vi "Run Framework.vi"(5 "components directory":path, 7 "framework options":T18={"FIFO Options"={"Infinite Timeouts"=FALSE}, "Thread Options"={"Show FP On Call"=TRUE, "Close FP After Call"=TRUE, "Allow Debugging"=TRUE}, "Plugin Options"={"Default Components"=TRUE}, "Performance Options"={"Measure Period"=TRUE, "Measure Rx/Tx Duration"=TRUE}, "Data Server Options"={"Enable Data Server"=FALSE, "Period"=50}} {"Data Server Options"."Period" format="%d ms"}, 8 "error in (no error)":errorcluster, 9 "thread settings":cluster{"Processor":i32, "Priority":i32}={"Processor"=-2, "Priority"=100}, 10 "framework configuration":T2, 11 "user interface pointers (null)":T1) -> (0 "error out":errorcluster)   [LabVIEW 2020]
uses:
  Includes/DSF Core.lvlibp/Classes/Framework/Framework Options.ctl
  Includes/DSF Core.lvlibp/Typedefs/DSF FIFO Options.ctl
  Includes/DSF Core.lvlibp/Classes/Thread/Thread Options.ctl
  Includes/DSF Core.lvlibp/Typedefs/DSF Plugin Options.ctl
  Includes/DSF Core.lvlibp/Typedefs/DSF Performance Options.ctl
  Includes/DSF Core.lvlibp/Classes/Framework/Data Server Options.ctl
  Includes/DSF Core.lvlibp/Typedefs/DSF Engine Framework Configuration.ctl
  Includes/DSF Core.lvlibp/Typedefs/DSF Engine Plugin Configuration.ctl
  Includes/DSF Core.lvlibp/Typedefs/Core Plugin Configuration.ctl
  Includes/DSF Core.lvlibp/Typedefs/DSF Timing Info.ctl
  Includes/DSF Core.lvlibp/Typedefs/DSF Settings Info.ctl
  Includes/DSF Core.lvlibp/Typedefs/DSF Engine Plugin Thread Configuration.ctl
  Includes/DSF Core.lvlibp/Typedefs/Core Thread Configuration.ctl
  Includes/DSF Core.lvlibp/Typedefs/DSF Engine Transfer Group Configuration.ctl
  Includes/DSF Core.lvlibp/Typedefs/Core Group Configuration.ctl
  Includes/DSF Core.lvlibp/Typedefs/DSF Direction.ctl
  Includes/DSF Core.lvlibp/Typedefs/DSF Timeout Behavior.ctl
  Includes/DSF Core.lvlibp/Typedefs/DSF Engine Transfer Configuration.ctl
  Includes/DSF Core.lvlibp/Typedefs/Core Transfer Configuration.ctl
  Includes/DSF Core.lvlibp/Typedefs/DSF Engine Channel Configuration.ctl
  Includes/DSF Core.lvlibp/Typedefs/Core Channel Configuration.ctl
  Includes/DSF Core.lvlibp/Typedefs/DSF Data Type.ctl
  SubVIs/UI Pointers.ctl
  <vilib>/NI/Memory Manager/Classes/Pointer/Pointer.lvclass
  <vilib>/NI/Memory Manager/Classes/Pointer/Pointer.lvclass/Pointer.ctl
  <vilib>/Platform/TimedLoop/XDataNode/timing_clust.ctl
  <vilib>/Platform/TimedLoop/XDataNode/nitl_modes.ctl
  <vilib>/Platform/TimedLoop/XDataNode/wakeup.ctl
  <vilib>/NI/Memory Manager/Classes/Pointer/Write U32.vi
  <vilib>/NI/Memory Manager/Classes/Pointer/Read U32.vi
  <vilib>/NI/Memory Manager/Classes/Pointer/Read I32.vi
  <vilib>/NI/Memory Manager/Classes/Pointer/Read Bool.vi
  <vilib>/NI/Memory Manager/Classes/Pointer/Write Bool.vi
  <vilib>/NI/Memory Manager/Classes/Pointer/Write I32.vi
  <vilib>/NI/Memory Manager/Classes/Pointer/Set Address.vi
  <vilib>/NI/Memory Manager/Classes/Pointer/Set Size.vi
  <vilib>/NI/Memory Manager/Classes/Pointer/Set Internal.vi
  <vilib>/NI/Memory Manager/Classes/Pointer/Check Null Pointer.vi
  <vilib>/NI/Memory Manager/Classes/Pointer/Clear (No Check).vi
  <vilib>/NI/Memory Manager/Classes/Pointer/Check Length.vi
  <vilib>/NI/Memory Manager/Classes/Pointer/Write (No Check).vi
  <vilib>/NI/Memory Manager/Classes/Pointer/Write (No Check) U32.vi
  <vilib>/NI/Memory Manager/Classes/Pointer/Check Move.vi
  <vilib>/NI/Memory Manager/Classes/Pointer/Read (No Check).vi
  <vilib>/NI/Memory Manager/Classes/Pointer/Read (No Check) U32.vi
  <vilib>/NI/Memory Manager/Classes/Pointer/Read (No Check) I32.vi
  <vilib>/NI/Memory Manager/Classes/Pointer/Read (No Check) Bool.vi
  <vilib>/NI/Memory Manager/Classes/Pointer/Write (No Check) Bool.vi
  <vilib>/NI/Memory Manager/Classes/Pointer/Write (No Check) I32.vi
  <vilib>/NI/Memory Manager/Classes/Pointer/Get Internal.vi
  <vilib>/NI/Memory Manager/Classes/Pointer/Errors.vi
  <vilib>/NI/Memory Manager/Classes/Pointer/Zone.vi
  <vilib>/NI/Memory Manager/Classes/Pointer/Null Pointer.vi
  <vilib>/NI/Memory Manager/Classes/Pointer/Check Bounds (Pointer).vi
  <vilib>/NI/Memory Manager/Classes/Pointer/Check Count.vi
  <vilib>/NI/Memory Manager/Classes/Pointer/Check Bounds (Power of 2).vi
  <vilib>/NI/Memory Manager/Classes/Pointer/Create Error.vi
  <vilib>/NI/Memory Manager/Classes/Pointer/Out of Bounds.vi
  <vilib>/NI/Memory Manager/Classes/Pointer/Check Bounds.vi
  <vilib>/NI/Memory Manager/VIs/New Error Cluster.vi
  <vilib>/NI/Memory Manager/VIs/New Error Cluster (512B).vi
  <vilib>/NI/Memory Manager/VIs/Set Error Status.vi
  <vilib>/NI/Memory Manager/VIs/Set Error Code.vi
  <vilib>/NI/Memory Manager/VIs/Set Error Source.vi
  <vilib>/NI/Memory Manager/Constants/Constants.vi
  <vilib>/NI/Memory Manager/Constants/Library Name.vi
  <vilib>/NI/Memory Manager/Classes/Pointer/Pointer Error Info.vi
  <vilib>/NI/Memory Manager/VIs/Write String to Source.vi
  <vilib>/NI/Memory Manager/Constants/Pointer Class Name.vi
  <vilib>/NI/Memory Manager/Classes/Pointer/Write Pointer Size to Error.vi
  <vilib>/NI/Memory Manager/VIs/Write Numeric to Source.vi
  <vilib>/NI/Memory Manager/VIs/Write Numeric Scalar to Source (Base10 U64).vi
  <vilib>/NI/Memory Manager/Classes/Pointer/Check Bounds (Buffer).vi
  <vilib>/NI/Memory Manager/Classes/Pointer/Buffer Underflow.vi
  Includes/DSF Core.lvlibp/Classes/Framework/Framework.lvclass
  <vilib>/platform/TimedLoop/XDataNode/XDataNode.xnode
  <vilib>/Platform/TimedLoop/XDataNode/XDNodeRunTimeDep.lvlib
  Includes/DSF Core.lvlibp/Classes/Configuration/Core/Framework/Framework Configuration.lvclass
  Includes/DSF Core.lvlibp
  Includes/DSF Core.lvlibp/Classes/Thread/Thread.lvclass
  Includes/DSF Core.lvlibp/Classes/Configuration/Core/Plugin/Plugin Configuration.lvclass
  Includes/DSF Core.lvlibp/Classes/Configuration/Core/Thread/Thread Configuration.lvclass
  Includes/DSF Core.lvlibp/Classes/Configuration/Core/Group/Group Configuration.lvclass
  Includes/DSF Core.lvlibp/Classes/Configuration/Core/Transfer/Transfer Configuration.lvclass
  Includes/DSF Core.lvlibp/Classes/Configuration/Core/Channel/Channel Configuration.lvclass
panel:
  out "actual frequency":u32 format="%.0pHz"
  in  "target frequency":u32=100 format="%.0pHz"
  out "iteration":i32
  in  "stop":bool
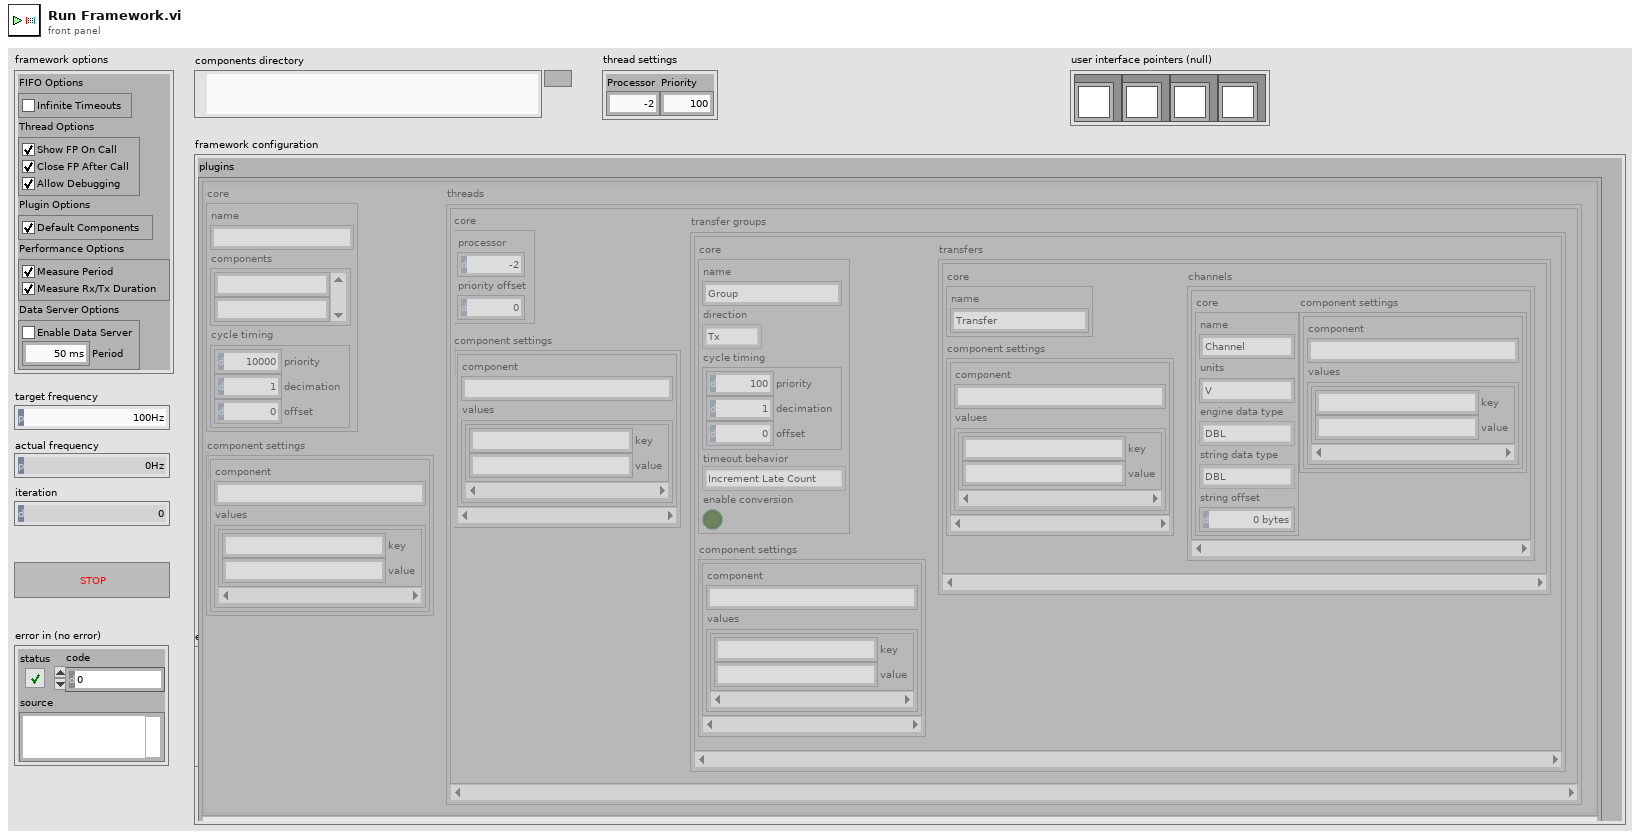
[diagram p1: front panel]
types:
  T1 = typedef "UI Pointers.ctl" = cluster{"Stop":refnum<class "Pointer.lvclass">, "Target Period":refnum<class "Pointer.lvclass">, "Actual Period":refnum<class "Pointer.lvclass">, "Iteration":refnum<class "Pointer.lvclass">}
  T2 = typedef "DSF Core.lvlibp/DSF Engine Framework Configuration.ctl" = cluster{"plugins":T3[]}
  T3 = typedef "DSF Core.lvlibp/DSF Engine Plugin Configuration.ctl" = cluster{"core":T4, "component settings":T6[], "threads":T7[]}
  T4 = typedef "DSF Core.lvlibp/Plugin Configuration.lvclass/Core Plugin Configuration.ctl" = cluster{"name":string, "components":string[], "cycle timing":T5}
  T5 = typedef "DSF Core.lvlibp/DSF Timing Info.ctl" = cluster{"priority":u64, "decimation":u64, "offset":u64}
  T6 = typedef "DSF Core.lvlibp/DSF Settings Info.ctl" = cluster{"component":string, "values":cluster{"key":string, "value":string}[]}
  T7 = typedef "DSF Core.lvlibp/DSF Engine Plugin Thread Configuration.ctl" = cluster{"core":T8, "component settings":T6[], "transfer groups":T9[]}
  T8 = typedef "DSF Core.lvlibp/Thread Configuration.lvclass/Core Thread Configuration.ctl" = cluster{"processor":i32, "priority offset":i16}
  T9 = typedef "DSF Core.lvlibp/DSF Engine Transfer Group Configuration.ctl" = cluster{"core":T10, "component settings":T6[], "transfers":T13[]}
  T10 = typedef "DSF Core.lvlibp/Group Configuration.lvclass/Core Group Configuration.ctl" = cluster{"name":string, "direction":T11, "cycle timing":T5, "timeout behavior":T12, "enable conversion":bool}
  T11 = typedef "DSF Core.lvlibp/DSF Direction.ctl" = enum8{"Tx", "Rx"}
  T12 = typedef "DSF Core.lvlibp/DSF Timeout Behavior.ctl" = enum8{"Increment Late Count", "Throw Error"}
  T13 = typedef "DSF Core.lvlibp/DSF Engine Transfer Configuration.ctl" = cluster{"core":T14, "component settings":T6[], "channels":T15[]}
  T14 = typedef "DSF Core.lvlibp/Transfer Configuration.lvclass/Core Transfer Configuration.ctl" = cluster{"name":string}
  T15 = typedef "DSF Core.lvlibp/DSF Engine Channel Configuration.ctl" = cluster{"core":T16, "component settings":T6[]}
  T16 = typedef "DSF Core.lvlibp/Channel Configuration.lvclass/Core Channel Configuration.ctl" = cluster{"name":string, "units":string, "engine data type":T17, "string data type":T17, "string offset":u64}
  T17 = typedef "DSF Core.lvlibp/DSF Data Type.ctl" = enum8{"Bool", "SGL", "DBL", "I8", "I16", "I32", "I64", "U8", "U16", "U32", "U64"}
  T18 = typedef "DSF Core.lvlibp/Framework.lvclass/Framework Options.ctl" = cluster{"FIFO Options":T19, "Thread Options":T20, "Plugin Options":T21, "Performance Options":T22, "Data Server Options":T23}
  T19 = typedef "DSF Core.lvlibp/Framework.lvclass/DSF FIFO Options.ctl" = cluster{"Infinite Timeouts":bool}
  T20 = typedef "DSF Core.lvlibp/Thread.lvclass/Thread Options.ctl" = cluster{"Show FP On Call":bool, "Close FP After Call":bool, "Allow Debugging":bool}
  T21 = typedef "DSF Core.lvlibp/Framework.lvclass/DSF Plugin Options.ctl" = cluster{"Default Components":bool}
  T22 = typedef "DSF Core.lvlibp/DSF Performance Options.ctl" = cluster{"Measure Period":bool, "Measure Rx/Tx Duration":bool}
  T23 = typedef "DSF Core.lvlibp/Framework.lvclass/Data Server Options.ctl" = cluster{"Enable Data Server":bool, "Period":u32}
  T24 = typedef "XDNodeRunTimeDep.lvlib/timing_clust.ctl" = cluster{"Expected End [f-1]":u64, "Actual End [f-1]":u64, "Finished Late? [f-1]":bool, "Expected End [i-1]":u64, "Actual End [i-1]":u64, "Finished Late? [i-1]":bool, "Expected Start [i]":u64, "Actual Start [i]":u64, "Expected Start [f]":u64, "Actual Start [f]":u64, "Source Name":string, "Structure Name":string, "Period":i64, "Deadline":i64, "Offset":i64, "Start":i64, "Priority":i32, "Timeout":i32, "Mode":T25, "Wakeup Reason":T26, "Error":errorcluster, "Source Type":string, "Secondary Source Type":string, "Global End Time":u64, "Global Start Time":u64, "Frame Duration":u64, "Iteration Duration":u64, "Assigned CPU":i32, "I/O Scan Engine Mode":u32}
  T25 = typedef "XDNodeRunTimeDep.lvlib/nitl_modes.ctl" = enum32{"No Change", "Process missed periods, maintain original phase", "Discard missed periods, maintain original phase", "Process missed periods, ignore original phase", "Discard missed periods, ignore original phase"}
  T26 = typedef "XDNodeRunTimeDep.lvlib/wakeup.ctl" = enum32{"Normal", "Aborted", "Asynchronous wakeup", "Timing source error", "Timed loop error", "Timeout"}
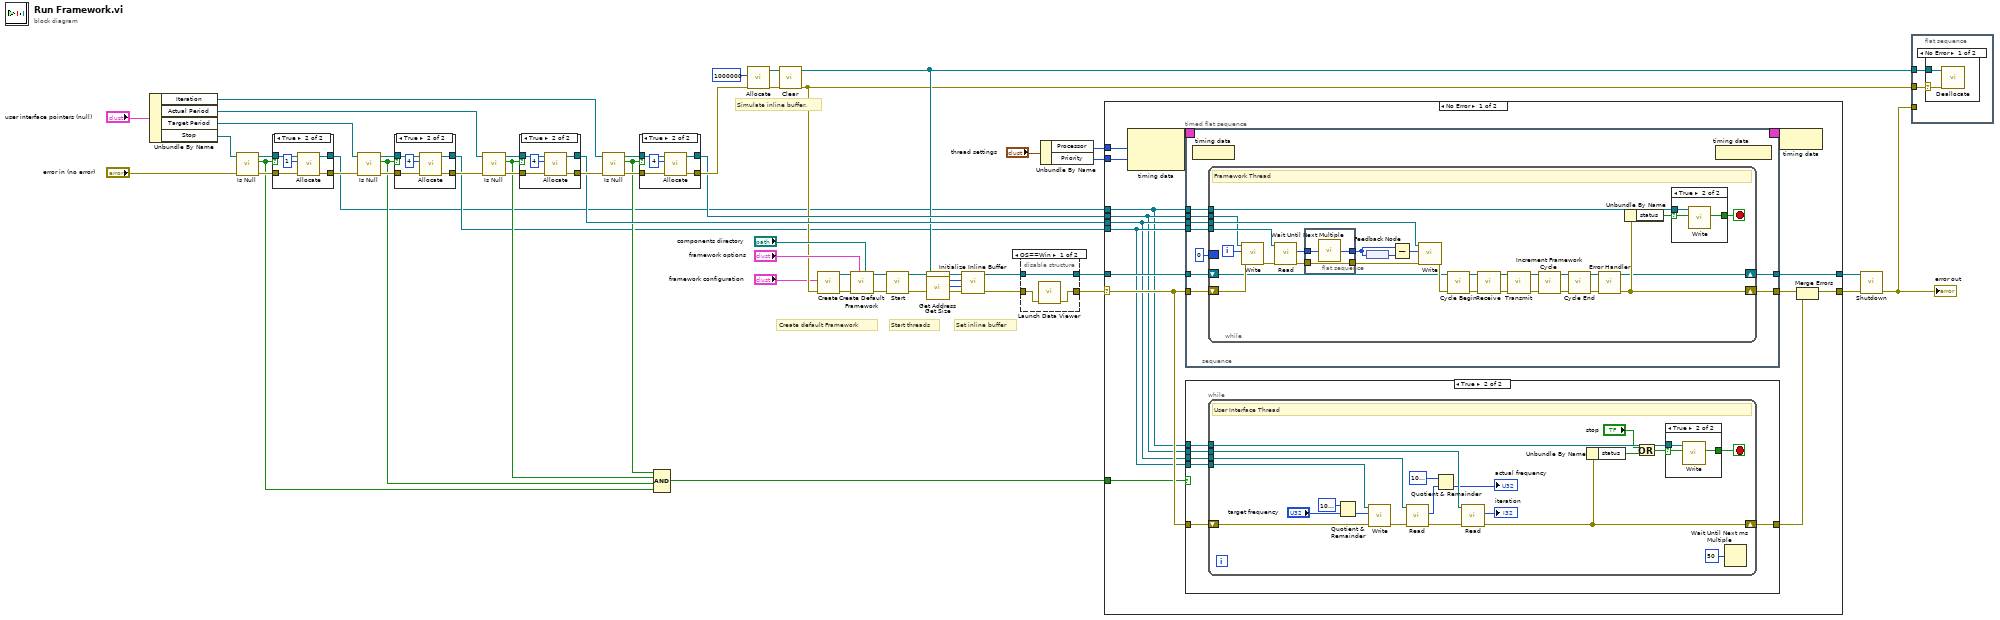
[diagram p0: block diagram]
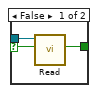
[diagram p5: hidden frame]
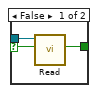
[diagram p6: hidden frame]
diagram:
  # "Set inline buffer"
  # "Start threads"
  # "Create default Framework"
  # "Simulate inline buffer."
  n1 = Unbundle By Name("user interface pointers (null)") -> ("Iteration"=w21:refnum<class "Pointer.lvclass">, "Actual Period"=w25:refnum<class "Pointer.lvclass">, "Target Period"=w29:refnum<class "Pointer.lvclass">, "Stop"=w35:refnum<class "Pointer.lvclass">)
  n2 = call <vilib>:"Is Null.vi"("error in (no error)"="error in (no error)", "Pointer in"=w35) -> ("error out"=w33:errorcluster, "null?"=w11:bool, "Pointer out"=w34:refnum<class "Pointer.lvclass">)  [unwired: 7 in]
  n3 = case shown="True" w11 {
    tunnel: w34 -> [w55 w59]
    tunnel: w33 -> [w54 w58]
    tunnel: [w55 w57] -> w1
    tunnel: [w54 w56] -> w30
    frame False {
    }
    frame True {
      n4 = call <vilib>:"Allocate.vi"("error in (no error)"=w58, "size"=u64 1, "Pointer type"=w59) -> ("error out"=w56:errorcluster, "Pointer out"=w57:refnum<class "Pointer.lvclass">)  [unwired: 7 in]
    }
  }
  n5 = call <vilib>:"Is Null.vi"("error in (no error)"=w30, "Pointer in"=w29) -> ("error out"=w31:errorcluster, "null?"=w10:bool, "Pointer out"=w32:refnum<class "Pointer.lvclass">)  [unwired: 7 in]
  n6 = case shown="True" w10 {
    tunnel: w32 -> [w62 w66]
    tunnel: w31 -> [w61 w65]
    tunnel: [w62 w64] -> w2
    tunnel: [w61 w63] -> w26
    frame False {
    }
    frame True {
      n7 = call <vilib>:"Allocate.vi"("error in (no error)"=w65, "size"=u64 4, "Pointer type"=w66) -> ("error out"=w63:errorcluster, "Pointer out"=w64:refnum<class "Pointer.lvclass">)  [unwired: 7 in]
    }
  }
  n8 = call <vilib>:"Is Null.vi"("error in (no error)"=w26, "Pointer in"=w25) -> ("error out"=w27:errorcluster, "null?"=w9:bool, "Pointer out"=w28:refnum<class "Pointer.lvclass">)  [unwired: 7 in]
  n9 = case shown="True" w9 {
    tunnel: w28 -> [w69 w73]
    tunnel: w27 -> [w68 w72]
    tunnel: [w69 w71] -> w17
    tunnel: [w68 w70] -> w22
    frame False {
    }
    frame True {
      n10 = call <vilib>:"Allocate.vi"("error in (no error)"=w72, "size"=u64 4, "Pointer type"=w73) -> ("error out"=w70:errorcluster, "Pointer out"=w71:refnum<class "Pointer.lvclass">)  [unwired: 7 in]
    }
  }
  n11 = call <vilib>:"Is Null.vi"("error in (no error)"=w22, "Pointer in"=w21) -> ("error out"=w23:errorcluster, "null?"=w8:bool, "Pointer out"=w24:refnum<class "Pointer.lvclass">)  [unwired: 7 in]
  n12 = case shown="True" w8 {
    tunnel: w24 -> [w76 w80]
    tunnel: w23 -> [w75 w79]
    tunnel: [w76 w78] -> w18
    tunnel: [w75 w77] -> w20
    frame False {
    }
    frame True {
      n13 = call <vilib>:"Allocate.vi"("error in (no error)"=w79, "size"=u64 4, "Pointer type"=w80) -> ("error out"=w77:errorcluster, "Pointer out"=w78:refnum<class "Pointer.lvclass">)  [unwired: 7 in]
    }
  }
  n14 = Compound Arithmetic op=AND(w8, w9, w10, w11) -> (w7:bool)
  n15 = call <vilib>:"Allocate.vi"("error in (no error)"=w20, "size"=u64 1000000) -> ("error out"=w49:errorcluster, "Pointer out"=w46:refnum<class "Pointer.lvclass">)  [unwired: 8 in]
  n16 = call <vilib>:"Clear.vi"("error in (no error)"=w49, "Pointer in"=w46) -> ("error out"=w6:errorcluster, "Pointer out"=w16:refnum<class "Pointer.lvclass">)  [unwired: 8 in]
  n17 = call "Create.vi"("error in (no error)"=w6, "framework configuration"="framework configuration") -> ("error out"=w5:errorcluster, "Framework Configuration out"=w4:refnum<class "Framework Configuration.lvclass">)  [unwired: 8 in]
  n18 = call "Create Default Framework.vi"("components directory (default)"="components directory", "framework options"="framework options", "error in (no error)"=w5, "Framework Configuration"=w4) -> ("error out"=w41:errorcluster, "Framework"=w45:refnum<class "Framework.lvclass">)  [unwired: 6 in]
  n19 = call-dynamic "Start.vi"("error in (no error)"=w41, "Framework in"=w45) -> ("error out"=w44:errorcluster, "Framework out"=w53:refnum<class "Framework.lvclass">)  [unwired: 8 in]
  n20 = call <vilib>:"Get Address.vi"("Pointer in"=w16) -> ("address"=w47:u64)  [unwired: 9 in, 1 out]
  n21 = call <vilib>:"Get Size.vi"("Pointer in"=w16) -> ("size"=w48:u64)  [unwired: 9 in, 1 out]
  n22 = call "Initialize Inline Buffer.vi"("error in (no error)"=w44, "size"=w48, "address"=w47, "Framework in"=w53) -> ("error out"=w42:errorcluster, "Framework out"=w43:refnum<class "Framework.lvclass">)  [unwired: 6 in]
  n23 = disable-structure shown="OS==Win" {
    disable-tunnel: [w84 w86] -> w39
    disable-tunnel: [w82 w85] -> w19
    disable-tunnel: w43 -> [w84 w86]
    disable-tunnel: w42 -> [w83 w85]
    frame condition #0 (active) {
      n24 = call "Launch Data Viewer.vi"("error in (no error)"=w83) -> ("error out"=w82:errorcluster)  [unwired: 10 in]
    }
    frame condition #1 {
    }
  }
  n25 = Unbundle By Name("thread settings") -> ("Processor"=w13:i32, "Priority"=w14:i32)
  n26 = case shown="No Error" w19 {
    selector: w19 -> [w101 w197]
    tunnel: [w94 w197] -> w52
    tunnel: w39 -> [w100 w198]
    tunnel: [w98 w198] -> w51
    tunnel: w1 -> [w91 _]
    tunnel: w2 -> [w99 _]
    tunnel: w17 -> [w93 _]
    tunnel: w18 -> [w92 _]
    tunnel: w13 -> [w90 _]
    tunnel: w14 -> [w89 _]
    tunnel: w7 -> [w88 _]
    frame No Error {
      n27 = node-c288(w90, w89) -> (w97:T24)
      n28 = timed-sequence {
        timing: w97 -> [_]
        timing-out: [_] -> w96
        tunnel: w100 -> [w142]
        tunnel: w101 -> [w141]
        tunnel: [w140] -> w98
        tunnel: [w139] -> w95
        tunnel: w91 -> [w138]
        tunnel: w99 -> [w137]
        tunnel: w93 -> [w136]
        tunnel: w92 -> [w135]
        n29 = timed-flat-sequence {
          tunnel: w142 -> [w151]
          tunnel: w141 -> [w150]
          tunnel: [w149] -> w140
          tunnel: [w148] -> w139
          tunnel: w138 -> [w147]
          tunnel: w137 -> [w146]
          tunnel: w136 -> [w145]
          tunnel: w135 -> [w144]
          n30 = node-c288() -> ()  [unwired: 1 in]
          n31 = while {
            shift-right: [w170] -> w149
            shift-left: w151 -> [w155]
            tunnel: w147 -> [w178]
            shift-right: [w173] -> w148
            shift-left: w150 -> [w159]
            tunnel: w146 -> [w171]
            tunnel: w145 -> [w161]
            tunnel: w144 -> [w158]
            border: u32 0 ("Tick Count(uSec)") -> [_]
            i -> [w163]
            stop <- w177 stop-if-true
            # "Framework Thread"
            n32 = call-poly <vilib>:"Write.vi"("error in (no error)"=w159, "value"=w163, "Pointer in"=w158) -> ("error out"=w160:errorcluster)  [unwired: 5 in, 3 out]
            n33 = call-poly <vilib>:"Read.vi"("error in (no error)"=w160, "Pointer in"=w171) -> ("error out"=w157:errorcluster, "value out"=w172:u32)  [unwired: 6 in, 2 out]
            n34 = flat-sequence {
              tunnel: w172 -> [w183]
              tunnel: [w182] -> w154
              tunnel: w157 -> [w181]
              tunnel: [w181] -> w156
              frame #0 {
                n35 = call "Wait Until Next Multiple"("Count(uSec)"=w183) -> ("Tick Count(uSec)"=w182:u32)
              }
            }
            n36 = feedback-in #1(w154) -> ()
            n37 = feedback #1() -> (w152:u32)
            n38 = Subtract(x=w154, y=w152) -> (x-y=w153:u32)
            n39 = call-poly <vilib>:"Write.vi"("error in (no error)"=w156, "value"=w153, "Pointer in"=w161) -> ("error out"=w162:errorcluster)  [unwired: 5 in, 3 out]
            n40 = call "Cycle Begin.vi"("error in (no error)"=w162, "Framework in"=w155) -> ("error out"=w175:errorcluster, "Framework out"=w176:refnum<class "Framework.lvclass">)  [unwired: 8 in]
            n41 = call "Receive.vi"("error in"=w175, "framework in"=w176) -> ("error out"=w180:errorcluster, "framework out"=w179:refnum<class "Framework.lvclass">)  [unwired: 8 in]
            n42 = call "Transmit.vi"("error in"=w180, "framework in"=w179) -> ("error out"=w169:errorcluster, "framework out"=w168:refnum<class "Framework.lvclass">)  [unwired: 8 in]
            n43 = call "Increment Framework Cycle.vi"("error in (no error)"=w169, "Framework in"=w168) -> ("error out"=w166:errorcluster, "Framework out"=w167:refnum<class "Framework.lvclass">)  [unwired: 8 in]
            n44 = call "Cycle End.vi"("error in (no error)"=w166, "Framework in"=w167) -> ("error out"=w165:errorcluster, "Framework out"=w164:refnum<class "Framework.lvclass">)  [unwired: 8 in]
            n45 = call "Error Handler.vi"("error in (no error)"=w165, "Framework in"=w164) -> ("error out"=w173:errorcluster, "Framework out"=w170:refnum<class "Framework.lvclass">)  [unwired: 8 in]
            n46 = Unbundle By Name(w173) -> ("status"=w174:bool)
            n47 = case shown="True" w174 {
              selector: w174 -> [w185 w188]
              tunnel: w178 -> [w186 w189]
              tunnel: [w184 w187] -> w177
              frame False {
                n48 = call-poly <vilib>:"Read.vi"("value in"=w185, "Pointer in"=w186) -> ("value out"=w184:bool)  [unwired: 6 in, 3 out]
              }
              frame True {
                n49 = call-poly <vilib>:"Write.vi"("value"=w188, "Pointer in"=w189) -> ("value"=w187:bool)  [unwired: 6 in, 3 out]
              }
            }
          }
          n50 = node-c288() -> ()  [unwired: 1 out]
        }
      }
      n51 = case shown="True" w88 {
        tunnel: w101 -> [w102 w108]
        tunnel: w99 -> [_ w107]
        tunnel: [w102 w106] -> w87
        tunnel: w93 -> [_ w105]
        tunnel: w92 -> [_ w104]
        tunnel: w91 -> [_ w103]
        frame False {
        }
        frame True {
          n52 = while {
            tunnel: w103 -> [w128]
            shift-right: [w115] -> w106
            shift-left: w108 -> [w123]
            tunnel: w107 -> [w119]
            tunnel: w105 -> [w117]
            tunnel: w104 -> [w113]
            stop <- w127 stop-if-true
            # "User Interface Thread"
            n53 = Quotient & Remainder(x=u32 1000000 ("y"), y="target frequency") -> (floor(x/y)=w118:u32)  [unwired: 1 out]
            n54 = call-poly <vilib>:"Write.vi"("error in (no error)"=w123, "value"=w118, "Pointer in"=w119) -> ("error out"=w120:errorcluster)  [unwired: 5 in, 3 out]
            n55 = call-poly <vilib>:"Read.vi"("error in (no error)"=w120, "Pointer in"=w117) -> ("error out"=w116:errorcluster, "value out"=w109:u32)  [unwired: 6 in, 2 out]
            n56 = Quotient & Remainder(x=u32 1000000 ("y"), y=w109) -> (floor(x/y)=→"actual frequency":u32)  [unwired: 1 out]
            n57 = call-poly <vilib>:"Read.vi"("error in (no error)"=w116, "Pointer in"=w113) -> ("error out"=w115:errorcluster, "value out"=→"iteration":i32)  [unwired: 6 in, 2 out]
            n58 = Unbundle By Name(w115) -> ("status"=w125:bool)
            n59 = Or(x="stop", y=w125) -> (x .or. y?=w126:bool)
            n60 = case shown="True" w126 {
              selector: w126 -> [w130 w133]
              tunnel: w128 -> [w131 w134]
              tunnel: [w129 w132] -> w127
              frame False {
                n61 = call-poly <vilib>:"Read.vi"("value in"=w130, "Pointer in"=w131) -> ("value out"=w129:bool)  [unwired: 6 in, 3 out]
              }
              frame True {
                n62 = call-poly <vilib>:"Write.vi"("value"=w133, "Pointer in"=w134) -> ("value"=w132:bool)  [unwired: 6 in, 3 out]
              }
            }
            n63 = Wait Until Next ms Multiple(millisecond multiple=u32 50) -> ()  [unwired: 1 out]
          }
        }
      }
      n64 = node-c288(w96) -> ()
      n65 = Merge Errors(w95, w87) -> (w94:errorcluster)
    }
    frame Error {
    }
  }
  n66 = call-dynamic "Shutdown.vi"("error in (no error)"=w52, "Framework in"=w51) -> ("error out"=w40:errorcluster)  [unwired: 8 in, 1 out]
  "error out" <- w40
  n67 = flat-sequence {
    tunnel: w16 -> [w200]
    tunnel: w40 -> [_]
    tunnel: w6 -> [w199]
    frame #0 {
      n68 = case shown="No Error" w199 {
        selector: w199 -> [w201 _]
        tunnel: w200 -> [w202 _]
        frame No Error {
          n69 = call <vilib>:"Deallocate.vi"("error in (no error)"=w201, "Pointer"=w202) -> ()  [unwired: 8 in, 2 out]
        }
        frame Error {
        }
      }
    }
  }
